vi "Get Resource ID.vi"(11 "Resource in":refnum<class "Resource.lvclass">) -> (2 "Resource ID":string)   [LabVIEW 2020, in "CTI.lvlib" / "Resource.lvclass"]
uses:
  Resource.lvclass
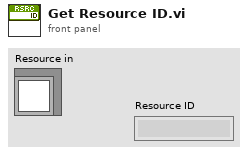
[diagram p1: front panel]
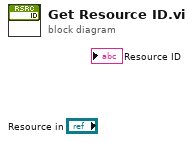
[diagram p0: block diagram]
diagram:
